vi "多路停止.vi"(0 "error in (no error)":errorcluster caption="错误输入（无错误）", 2 "停止1":bool, 3 "停止":bool, 4 "停止2":bool) -> (7 "error in (no error)":errorcluster caption="错误输入（无错误）", 9 "为假停止":bool, 10 "为真停止":bool)   [LabVIEW 2013]
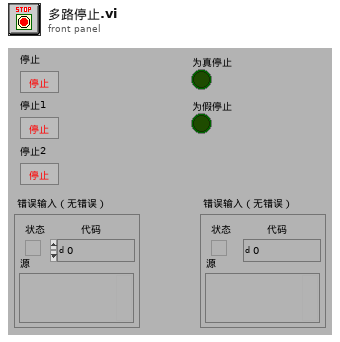
[diagram p1: front panel]
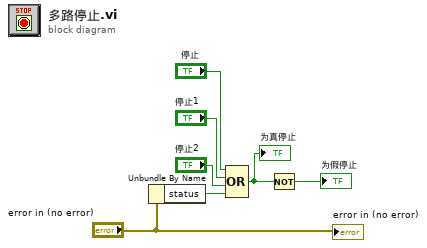
[diagram p0: block diagram]
diagram:
  n1 = Unbundle By Name("error in (no error)") -> ("status"=w4:bool)
  n2 = Compound Arithmetic op=OR("停止", "停止1", "停止2", w4) -> (w2:bool)
  "为真停止" <- w2
  n3 = Not(x=w2) -> (.not. x?=→"为假停止":bool)
  "error in (no error)" <- "error in (no error)"
